vi "checkColors.vi"(10 "Colors [4]":cluster{u32, u32}[](array[cluster]), 11 "Array":cluster{u32, u32}[](array[cluster])) -> (3 "Boolean":bool)   [LabVIEW 2014]
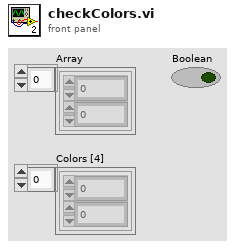
[diagram p1: front panel]
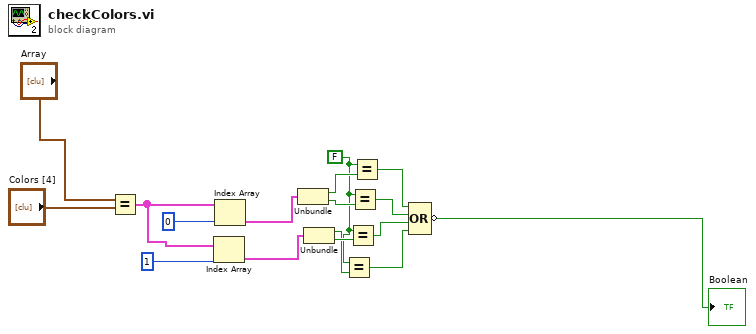
[diagram p0: block diagram]
diagram:
  w6 = FALSE
  n1 = Equal?(x="Array", y="Colors [4]") -> (x = y?=w15:cluster{bool, bool}[])
  n2 = Index Array(array=w15, index=1) -> (element=w17:cluster{bool, bool})
  n3 = Index Array(array=w15, index=0) -> (element=w13:cluster{bool, bool})
  n4 = Unbundle(w13) -> (w8:bool, w9:bool)
  n5 = Unbundle(w17) -> (w7:bool, w12:bool)
  n6 = Equal?(x=w6, y=w7) -> (x = y?=w2:bool)
  n7 = Equal?(x=w6, y=w12) -> (x = y?=w3:bool)
  n8 = Equal?(x=w6, y=w9) -> (x = y?=w4:bool)
  n9 = Equal?(x=w6, y=w8) -> (x = y?=w5:bool)
  n10 = Compound Arithmetic op=OR(w5, w4, w3, w2) -> (invert →"Boolean":bool)
